vi "S4GUI_001.vi"() -> ()   [LabVIEW 2018] (continued)
            n3363 = call "Write target.vi"("error in (no error)"=w8575, "target"=0.0, "Optics in"=w8577) -> ("error out"=w8574:errorcluster, "Optics out"=w8578:refnum<class "Opt_Selector.lvclass">)  [unwired: 7 in]
            n3364 = call "Write target name.vi"("error in (no error)"=w8574, "target name"=w8568, "Optics in"=w8578) -> ("error out"=w8573:errorcluster, "Optics out"=w8579:refnum<class "Opt_Selector.lvclass">)  [unwired: 7 in]
            n3365 = call "Write CALW.vi"("error in (no error)"=w8573, "Opt_Selector.lvclass"=w8579, "Instrument in"=w8576) -> ("error out"=w8563:errorcluster, "Instrument out"=w8571:refnum<class "Instrument.lvclass">)  [unwired: 7 in]
            n3366 = property on="Calibrator Selector" class="Ring (strict)"(error in=w8563, "Value"=w8562, "DisabledEnum"=T7."Disabled and Grayed Out" ("Disabled")) -> (error out=w8565:errorcluster)  [unwired: 1 in, 1 out]
            n3367 = property on="Calibrator Selector" class="Ring (strict)"(error in=w8565, "RingText.Text"="OFF" ("Ring Text.Text")) -> (error out=w8564:errorcluster)  [unwired: 1 in, 1 out]
            n3368 = case shown="True" w8560 {
              tunnel: [u8 0 ("SHUTTER_MODE") w8582] -> w8561
              tunnel: w8559 -> [_ w8581]
              frame False {
                # "Fotom. & Async"
                # "Internal"
              }
              frame True {
                # "Ext. Start"
                # "Internal"
                # "Fotom. Sync. SEM exp mode"
                # "Fotom. Sync. COM exp mode"
                n3369 = Select(t=u8 0, s=w8581, f=u8 6 ("SHUTTER_MODE")) -> (s? t:f=w8582:u8)
              }
            }
          }
          frame Default {
            # "Polar. COM exp mode"
            # "Internal"
            # "Polar. SEM exp mode"
            # "Ext. Start"
            n3370 = Select(t=u8 0, s=w8588, f=u8 6 ("SHUTTER_MODE")) -> (s? t:f=w8585:u8)
          }
        }
        n3371 = call "Write Instrument.lvclass.vi"("error in (no error)"=w8236, "Instrument.lvclass"=w8319, "S4ACS_GUI in"=w8220) -> ("error out"=w8235:errorcluster, "S4ACS_GUI out"=w8224:refnum<class "S4GUI.lvclass">)  [unwired: 7 in]
        n3372 = call-dynamic "Read AcquisitionC.vi"("error in (no error)"=w8235, "S4ACS_GUI in"=w8224) -> ("error out"=w8246:errorcluster, "Acquisition.lvclass"=w8245:refnum<class "Acquisition.lvclass">)  [unwired: 7 in, 1 out]
        n3373 = call-dynamic "Read AcquisitionA.vi"("error in (no error)"=w8235, "S4ACS_GUI in"=w8224) -> ("error out"=w8249:errorcluster, "Acquisition.lvclass"=w8250:refnum<class "Acquisition.lvclass">)  [unwired: 7 in, 1 out]
        n3374 = call "Read AcquisitionB.vi"("error in (no error)"=w8235, "S4ACS_GUI in"=w8224) -> ("error out"=w8247:errorcluster, "Acquisition.lvclass"=w8248:refnum<class "Acquisition.lvclass">)  [unwired: 7 in, 1 out]
        n3375 = call-dynamic "Read AcquisitionD.vi"("error in (no error)"=w8235, "S4ACS_GUI in"=w8224) -> ("error out"=w8243:errorcluster, "Acquisition.lvclass"=w8244:refnum<class "Acquisition.lvclass">)  [unwired: 7 in, 1 out]
        n3376 = call "Read connection.vi"("error in (no error)"=w8246, "Server in"=w8245) -> ("error out"=w8252:errorcluster, "connection"=w8251:bool, "Server out"=w8253:refnum<class "Acquisition.lvclass">)  [unwired: 7 in]
        n3377 = call "Read connection.vi"("error in (no error)"=w8247, "Server in"=w8248) -> ("error out"=w8255:errorcluster, "connection"=w8254:bool, "Server out"=w8256:refnum<class "Acquisition.lvclass">)  [unwired: 7 in]
        n3378 = call "Read connection.vi"("error in (no error)"=w8243, "Server in"=w8244) -> ("error out"=w8232:errorcluster, "connection"=w8233:bool, "Server out"=w8234:refnum<class "Acquisition.lvclass">)  [unwired: 7 in]
        n3379 = call "Read connection.vi"("error in (no error)"=w8249, "Server in"=w8250) -> ("error out"=w8258:errorcluster, "connection"=w8257:bool, "Server out"=w8259:refnum<class "Acquisition.lvclass">)  [unwired: 7 in]
        n3380 = case shown="True" w8251 {
          tunnel: w8253 -> [w8426 w8431]
          tunnel: w8252 -> [w8425 w8430]
          tunnel: [w8426 w8429] -> w8238
          tunnel: [w8425 w8428] -> w8237
          tunnel: w8231 -> [_ w8427]
          frame False {
          }
          frame True {
            # "nome do arquivo .cfg"
            # "seção no arquivo .cfg"
            n3381 = call-dynamic "Read Channel.vi"("error in (no error)"=w8430, "Acquisition in"=w8431) -> ("error out"=w8435:errorcluster, "Channel.lvclass"=w8434:refnum<class "Channel.lvclass">, "Acquisition out"=w8433:refnum<class "Acquisition.lvclass">)  [unwired: 7 in]
            n3382 = call-dynamic "Read Interface.vi"("error in (no error)"=w8435, "Channel in"=w8434) -> ("error out"=w8442:errorcluster, "Interface.lvclass"=w8443:refnum<class "Interface.lvclass">, "Channel out"=w8432:refnum<class "Channel.lvclass">)  [unwired: 7 in]
            n3383 = call-dynamic "Get CCD_Config.vi"("error in (no error)"=w8442, "Interface in"=w8443) -> ("error out"=w8440:errorcluster, "output cluster"=w8439:T24, "Interface out"=w8444:refnum<class "Interface.lvclass">)  [unwired: 7 in]
            n3384 = Bundle By Name(cluster=w8439, "TRIGGER_MODE"=w8427) -> (w8441:T24)
            n3385 = call-dynamic "Set CCD_Config.vi"("error in (no error)"=w8440, "input cluster"=w8441, "Interface in"=w8444) -> ("error out"=w8438:errorcluster, "Interface out"=w8445:refnum<class "Interface.lvclass">)  [unwired: 7 in]
            n3386 = Flatten To String(anything=w8441, error in (no error)=w8438) -> (data string=w8436:string, error out=w8437:errorcluster)  [unwired: 2 in, 1 out]
            n3387 = call "Write flatted cluster.vi"("error in (no error)"=w8437, "flatted cluster"=w8436, "Interface in"=w8445) -> ("error out"=w8447:errorcluster, "Interface out"=w8446:refnum<class "Interface.lvclass">)  [unwired: 7 in]
            n3388 = call-dynamic "Write Interface.vi"("error in (no error)"=w8447, "Interface.lvclass"=w8446, "Channel in"=w8432) -> ("error out"=w8453:errorcluster, "Channel out"=w8454:refnum<class "Channel.lvclass">)  [unwired: 7 in]
            n3389 = call "Write section_name.vi"("error in (no error)"=w8453, "section_name"="CCD_ACS3", "Channel in"=w8454) -> ("error out"=w8451:errorcluster, "Channel out"=w8457:refnum<class "Channel.lvclass">)  [unwired: 7 in]
            n3390 = call-dynamic "save config.vi"("error in (no error)"=w8451, "file config"="lastsaved.cfg", "Channel in"=w8457) -> ("error out"=w8452:errorcluster, "Channel out"=w8458:refnum<class "Channel.lvclass">)  [unwired: 7 in]
            n3391 = call-dynamic "Read State Machine.vi"("error in (no error)"=w8452, "Device in"=w8458) -> ("error out"=w8448:errorcluster, "State Machine.lvclass"=w8460:refnum<class "State Machine.lvclass">, "Device out"=w8459:refnum<class "Channel.lvclass">)  [unwired: 7 in]
            n3392 = call-dynamic "Write State.vi"("error in (no error)"=w8448, "State"=60, "State Machine in"=w8460) -> ("error out"=w8449:errorcluster, "State Machine out"=w8461:refnum<class "State Machine.lvclass">)  [unwired: 7 in]
            n3393 = call-dynamic "Write State Machine.vi"("error in (no error)"=w8449, "State Machine.lvclass"=w8461, "Device in"=w8459) -> ("error out"=w8463:errorcluster, "Device out"=w8462:refnum<class "Channel.lvclass">)  [unwired: 7 in]
            n3394 = call-dynamic "Write Channel.vi"("error in (no error)"=w8463, "Channel.lvclass"=w8462, "Acquisition in"=w8433) -> ("error out"=w8428:errorcluster, "Acquisition out"=w8429:refnum<class "Acquisition.lvclass">)  [unwired: 7 in]
          }
        }
        n3395 = case shown="True" w8233 {
          tunnel: w8234 -> [w8387 w8392]
          tunnel: w8232 -> [w8386 w8391]
          tunnel: w8231 -> [_ w8390]
          tunnel: [w8387 w8389] -> w8230
          tunnel: [w8386 w8388] -> w8229
          frame False {
          }
          frame True {
            # "nome do arquivo .cfg"
            # "seção no arquivo .cfg"
            n3396 = call-dynamic "Read Channel.vi"("error in (no error)"=w8391, "Acquisition in"=w8392) -> ("error out"=w8421:errorcluster, "Channel.lvclass"=w8422:refnum<class "Channel.lvclass">, "Acquisition out"=w8423:refnum<class "Acquisition.lvclass">)  [unwired: 7 in]
            n3397 = call-dynamic "Read Interface.vi"("error in (no error)"=w8421, "Channel in"=w8422) -> ("error out"=w8414:errorcluster, "Interface.lvclass"=w8413:refnum<class "Interface.lvclass">, "Channel out"=w8424:refnum<class "Channel.lvclass">)  [unwired: 7 in]
            n3398 = call-dynamic "Get CCD_Config.vi"("error in (no error)"=w8414, "Interface in"=w8413) -> ("error out"=w8416:errorcluster, "output cluster"=w8417:T24, "Interface out"=w8412:refnum<class "Interface.lvclass">)  [unwired: 7 in]
            n3399 = Bundle By Name(cluster=w8417, "TRIGGER_MODE"=w8390) -> (w8415:T24)
            n3400 = call-dynamic "Set CCD_Config.vi"("error in (no error)"=w8416, "input cluster"=w8415, "Interface in"=w8412) -> ("error out"=w8418:errorcluster, "Interface out"=w8411:refnum<class "Interface.lvclass">)  [unwired: 7 in]
            n3401 = Flatten To String(anything=w8415, error in (no error)=w8418) -> (data string=w8420:string, error out=w8419:errorcluster)  [unwired: 2 in, 1 out]
            n3402 = call "Write flatted cluster.vi"("error in (no error)"=w8419, "flatted cluster"=w8420, "Interface in"=w8411) -> ("error out"=w8409:errorcluster, "Interface out"=w8410:refnum<class "Interface.lvclass">)  [unwired: 7 in]
            n3403 = call-dynamic "Write Interface.vi"("error in (no error)"=w8409, "Interface.lvclass"=w8410, "Channel in"=w8424) -> ("error out"=w8403:errorcluster, "Channel out"=w8402:refnum<class "Channel.lvclass">)  [unwired: 7 in]
            n3404 = call "Write section_name.vi"("error in (no error)"=w8403, "section_name"="CCD_ACS4", "Channel in"=w8402) -> ("error out"=w8405:errorcluster, "Channel out"=w8399:refnum<class "Channel.lvclass">)  [unwired: 7 in]
            n3405 = call-dynamic "save config.vi"("error in (no error)"=w8405, "file config"="lastsaved.cfg", "Channel in"=w8399) -> ("error out"=w8404:errorcluster, "Channel out"=w8398:refnum<class "Channel.lvclass">)  [unwired: 7 in]
            n3406 = call-dynamic "Read State Machine.vi"("error in (no error)"=w8404, "Device in"=w8398) -> ("error out"=w8408:errorcluster, "State Machine.lvclass"=w8396:refnum<class "State Machine.lvclass">, "Device out"=w8397:refnum<class "Channel.lvclass">)  [unwired: 7 in]
            n3407 = call-dynamic "Write State.vi"("error in (no error)"=w8408, "State"=60, "State Machine in"=w8396) -> ("error out"=w8407:errorcluster, "State Machine out"=w8395:refnum<class "State Machine.lvclass">)  [unwired: 7 in]
            n3408 = call-dynamic "Write State Machine.vi"("error in (no error)"=w8407, "State Machine.lvclass"=w8395, "Device in"=w8397) -> ("error out"=w8393:errorcluster, "Device out"=w8394:refnum<class "Channel.lvclass">)  [unwired: 7 in]
            n3409 = call-dynamic "Write Channel.vi"("error in (no error)"=w8393, "Channel.lvclass"=w8394, "Acquisition in"=w8423) -> ("error out"=w8388:errorcluster, "Acquisition out"=w8389:refnum<class "Acquisition.lvclass">)  [unwired: 7 in]
          }
        }
        n3410 = case shown="True" w8254 {
          tunnel: w8256 -> [w8465 w8470]
          tunnel: w8255 -> [w8464 w8469]
          tunnel: [w8465 w8468] -> w8240
          tunnel: [w8464 w8467] -> w8239
          tunnel: w8231 -> [_ w8466]
          frame False {
          }
          frame True {
            # "nome do arquivo .cfg"
            # "seção no arquivo .cfg"
            n3411 = call-dynamic "Read Channel.vi"("error in (no error)"=w8469, "Acquisition in"=w8470) -> ("error out"=w8474:errorcluster, "Channel.lvclass"=w8473:refnum<class "Channel.lvclass">, "Acquisition out"=w8472:refnum<class "Acquisition.lvclass">)  [unwired: 7 in]
            n3412 = call-dynamic "Read Interface.vi"("error in (no error)"=w8474, "Channel in"=w8473) -> ("error out"=w8481:errorcluster, "Interface.lvclass"=w8482:refnum<class "Interface.lvclass">, "Channel out"=w8471:refnum<class "Channel.lvclass">)  [unwired: 7 in]
            n3413 = call-dynamic "Get CCD_Config.vi"("error in (no error)"=w8481, "Interface in"=w8482) -> ("error out"=w8479:errorcluster, "output cluster"=w8478:T24, "Interface out"=w8483:refnum<class "Interface.lvclass">)  [unwired: 7 in]
            n3414 = Bundle By Name(cluster=w8478, "TRIGGER_MODE"=w8466) -> (w8480:T24)
            n3415 = call-dynamic "Set CCD_Config.vi"("error in (no error)"=w8479, "input cluster"=w8480, "Interface in"=w8483) -> ("error out"=w8477:errorcluster, "Interface out"=w8484:refnum<class "Interface.lvclass">)  [unwired: 7 in]
            n3416 = Flatten To String(anything=w8480, error in (no error)=w8477) -> (data string=w8475:string, error out=w8476:errorcluster)  [unwired: 2 in, 1 out]
            n3417 = call "Write flatted cluster.vi"("error in (no error)"=w8476, "flatted cluster"=w8475, "Interface in"=w8484) -> ("error out"=w8486:errorcluster, "Interface out"=w8485:refnum<class "Interface.lvclass">)  [unwired: 7 in]
            n3418 = call-dynamic "Write Interface.vi"("error in (no error)"=w8486, "Interface.lvclass"=w8485, "Channel in"=w8471) -> ("error out"=w8492:errorcluster, "Channel out"=w8493:refnum<class "Channel.lvclass">)  [unwired: 7 in]
            n3419 = call "Write section_name.vi"("error in (no error)"=w8492, "section_name"="CCD_ACS2", "Channel in"=w8493) -> ("error out"=w8490:errorcluster, "Channel out"=w8496:refnum<class "Channel.lvclass">)  [unwired: 7 in]
            n3420 = call-dynamic "save config.vi"("error in (no error)"=w8490, "file config"="lastsaved.cfg", "Channel in"=w8496) -> ("error out"=w8491:errorcluster, "Channel out"=w8497:refnum<class "Channel.lvclass">)  [unwired: 7 in]
            n3421 = call-dynamic "Read State Machine.vi"("error in (no error)"=w8491, "Device in"=w8497) -> ("error out"=w8487:errorcluster, "State Machine.lvclass"=w8499:refnum<class "State Machine.lvclass">, "Device out"=w8498:refnum<class "Channel.lvclass">)  [unwired: 7 in]
            n3422 = call-dynamic "Write State.vi"("error in (no error)"=w8487, "State"=60, "State Machine in"=w8499) -> ("error out"=w8488:errorcluster, "State Machine out"=w8500:refnum<class "State Machine.lvclass">)  [unwired: 7 in]
            n3423 = call-dynamic "Write State Machine.vi"("error in (no error)"=w8488, "State Machine.lvclass"=w8500, "Device in"=w8498) -> ("error out"=w8502:errorcluster, "Device out"=w8501:refnum<class "Channel.lvclass">)  [unwired: 7 in]
            n3424 = call-dynamic "Write Channel.vi"("error in (no error)"=w8502, "Channel.lvclass"=w8501, "Acquisition in"=w8472) -> ("error out"=w8467:errorcluster, "Acquisition out"=w8468:refnum<class "Acquisition.lvclass">)  [unwired: 7 in]
          }
        }
        n3425 = case shown="True" w8257 {
          tunnel: [w8503 w8537] -> w8241
          tunnel: [w8504 w8536] -> w8242
          tunnel: w8259 -> [w8504 w8507]
          tunnel: w8258 -> [w8503 w8506]
          tunnel: w8231 -> [_ w8505]
          frame False {
          }
          frame True {
            # "nome do arquivo .cfg"
            # "seção no arquivo .cfg"
            n3426 = call-dynamic "Read Channel.vi"("error in (no error)"=w8506, "Acquisition in"=w8507) -> ("error out"=w8538:errorcluster, "Channel.lvclass"=w8539:refnum<class "Channel.lvclass">, "Acquisition out"=w8540:refnum<class "Acquisition.lvclass">)  [unwired: 7 in]
            n3427 = call-dynamic "Read Interface.vi"("error in (no error)"=w8538, "Channel in"=w8539) -> ("error out"=w8529:errorcluster, "Interface.lvclass"=w8528:refnum<class "Interface.lvclass">, "Channel out"=w8541:refnum<class "Channel.lvclass">)  [unwired: 7 in]
            n3428 = call-dynamic "Get CCD_Config.vi"("error in (no error)"=w8529, "Interface in"=w8528) -> ("error out"=w8531:errorcluster, "output cluster"=w8532:T24, "Interface out"=w8527:refnum<class "Interface.lvclass">)  [unwired: 7 in]
            n3429 = Bundle By Name(cluster=w8532, "TRIGGER_MODE"=w8505) -> (w8530:T24)
            n3430 = call-dynamic "Set CCD_Config.vi"("error in (no error)"=w8531, "input cluster"=w8530, "Interface in"=w8527) -> ("error out"=w8533:errorcluster, "Interface out"=w8526:refnum<class "Interface.lvclass">)  [unwired: 7 in]
            n3431 = Flatten To String(anything=w8530, error in (no error)=w8533) -> (data string=w8535:string, error out=w8534:errorcluster)  [unwired: 2 in, 1 out]
            n3432 = call "Write flatted cluster.vi"("error in (no error)"=w8534, "flatted cluster"=w8535, "Interface in"=w8526) -> ("error out"=w8524:errorcluster, "Interface out"=w8525:refnum<class "Interface.lvclass">)  [unwired: 7 in]
            n3433 = call-dynamic "Write Interface.vi"("error in (no error)"=w8524, "Interface.lvclass"=w8525, "Channel in"=w8541) -> ("error out"=w8519:errorcluster, "Channel out"=w8518:refnum<class "Channel.lvclass">)  [unwired: 7 in]
            n3434 = call "Write section_name.vi"("error in (no error)"=w8519, "section_name"="CCD_ACS1", "Channel in"=w8518) -> ("error out"=w8520:errorcluster, "Channel out"=w8515:refnum<class "Channel.lvclass">)  [unwired: 7 in]
            n3435 = call-dynamic "save config.vi"("error in (no error)"=w8520, "file config"="lastsaved.cfg", "Channel in"=w8515) -> ("error out"=w8508:errorcluster, "Channel out"=w8509:refnum<class "Channel.lvclass">)  [unwired: 7 in]
            n3436 = call-dynamic "Read State Machine.vi"("error in (no error)"=w8508, "Device in"=w8509) -> ("error out"=w8523:errorcluster, "State Machine.lvclass"=w8513:refnum<class "State Machine.lvclass">, "Device out"=w8514:refnum<class "Channel.lvclass">)  [unwired: 7 in]
            n3437 = call-dynamic "Write State.vi"("error in (no error)"=w8523, "State"=60, "State Machine in"=w8513) -> ("error out"=w8522:errorcluster, "State Machine out"=w8512:refnum<class "State Machine.lvclass">)  [unwired: 7 in]
            n3438 = call-dynamic "Write State Machine.vi"("error in (no error)"=w8522, "State Machine.lvclass"=w8512, "Device in"=w8514) -> ("error out"=w8510:errorcluster, "Device out"=w8511:refnum<class "Channel.lvclass">)  [unwired: 7 in]
            n3439 = call-dynamic "Write Channel.vi"("error in (no error)"=w8510, "Channel.lvclass"=w8511, "Acquisition in"=w8540) -> ("error out"=w8537:errorcluster, "Acquisition out"=w8536:refnum<class "Acquisition.lvclass">)  [unwired: 7 in]
          }
        }
        n3440 = call-dynamic "Write AcquisitionA.vi"("error in (no error)"=w8241, "Acquisition.lvclass"=w8242, "S4ACS_GUI in"=w8224) -> ("error out"=w8228:errorcluster, "S4ACS_GUI out"=w8223:refnum<class "S4GUI.lvclass">)  [unwired: 7 in]
        n3441 = call "Write AcquisitionB.vi"("error in (no error)"=w8239, "Acquisition.lvclass"=w8240, "S4ACS_GUI in"=w8223) -> ("error out"=w8227:errorcluster, "S4ACS_GUI out"=w8222:refnum<class "S4GUI.lvclass">)  [unwired: 7 in]
        n3442 = call-dynamic "Write AcquisitionC.vi"("error in (no error)"=w8237, "Acquisition.lvclass"=w8238, "S4ACS_GUI in"=w8222) -> ("error out"=w8226:errorcluster, "S4ACS_GUI out"=w8221:refnum<class "S4GUI.lvclass">)  [unwired: 7 in]
        n3443 = call-dynamic "Write AcquisitionD.vi"("error in (no error)"=w8229, "Acquisition.lvclass"=w8230, "S4ACS_GUI in"=w8221) -> ("error out"=w8225:errorcluster, "S4ACS_GUI out"=w8204:refnum<class "S4GUI.lvclass">)  [unwired: 7 in]
        n3444 = Merge Errors(w8228, w8227, w8226, w8225) -> (w8201:errorcluster)
        n3445 = call "Read Instrument.lvclass.vi"("error in (no error)"=w8201, "S4ACS_GUI in"=w8204) -> ("error out"=w8209:errorcluster, "Instrument.lvclass"=w8208:refnum<class "Instrument.lvclass">, "S4ACS_GUI out"=w8205:refnum<class "S4GUI.lvclass">)  [unwired: 7 in]
        n3446 = call "Read ASEL.vi"("error in (no error)"=w8209, "Instrument in"=w8208) -> ("error out"=w8217:errorcluster, "Opt_Selector.lvclass"=w8216:refnum<class "Opt_Selector.lvclass">, "Instrument out"=w8215:refnum<class "Instrument.lvclass">)  [unwired: 7 in]
        n3447 = call "Read target name.vi"("error in (no error)"=w8217, "Optics in"=w8216) -> ("error out"=w8213:errorcluster, "target name"=w8212:string, "Optics out"=w8214:refnum<class "Opt_Selector.lvclass">)  [unwired: 7 in]
        n3448 = call "Write ASEL.vi"("error in (no error)"=w8213, "Opt_Selector.lvclass"=w8214, "Instrument in"=w8215) -> ("error out"=w8211:errorcluster, "Instrument out"=w8207:refnum<class "Instrument.lvclass">)  [unwired: 7 in]
        n3449 = case shown="\"ON\"" w8212 {
          tunnel: w8211 -> [w8362 w8373]
          tunnel: [w8362 w8369] -> w8210
          tunnel: w8207 -> [w8361 w8374]
          tunnel: [w8361 w8370] -> w8206
          frame Default {
          }
          frame "ON" {
            n3450 = call "Read WPROT.vi"("error in (no error)"=w8373, "Instrument in"=w8374) -> ("error out"=w8365:errorcluster, "Opt_Selector.lvclass"=w8372:refnum<class "Opt_Selector.lvclass">, "Instrument out"=w8371:refnum<class "Instrument.lvclass">)  [unwired: 7 in]
            n3451 = call-dynamic "Read sequencia.vi"("error in (no error)"=w8365, "Opt_Selector in"=w8372) -> ("error out"=w8364:errorcluster, "sequencia"=w8368:u16, "Opt_Selector out"=w8367:refnum<class "Opt_Selector.lvclass">)  [unwired: 7 in]
            n3452 = case shown="0" w8368 {
              tunnel: w8367 -> [w8376 w8385]
              tunnel: [w8376 w8381] -> w8366
              tunnel: w8364 -> [w8375 w8384]
              tunnel: [w8375 w8379] -> w8363
              frame Default {
              }
              frame 0 {
                n3453 = call-dynamic "Write sequencia.vi"("error in (no error)"=w8384, "sequencia"=u16 1, "Opt_Selector in"=w8385) -> ("error out"=w8380:errorcluster, "Opt_Selector out"=w8382:refnum<class "Opt_Selector.lvclass">)  [unwired: 7 in]
                n3454 = local write "P0"(TRUE ("P0")) -> ()
                n3455 = call-dynamic "Write sequencia_ant.vi"("error in (no error)"=w8380, "sequencia_ant"=u16 1, "Opt_Selector in"=w8382) -> ("error out"=w8379:errorcluster, "Opt_Selector out"=w8381:refnum<class "Opt_Selector.lvclass">)  [unwired: 7 in]
              }
            }
            n3456 = call "Write WPROT.vi"("error in (no error)"=w8363, "Opt_Selector.lvclass"=w8366, "Instrument in"=w8371) -> ("error out"=w8369:errorcluster, "Instrument out"=w8370:refnum<class "Instrument.lvclass">)  [unwired: 7 in]
          }
        }
        n3457 = call "Write Instrument.lvclass.vi"("error in (no error)"=w8210, "Instrument.lvclass"=w8206, "S4ACS_GUI in"=w8205) -> ("error out"=w8202:errorcluster, "S4ACS_GUI out"=w8203:refnum<class "S4GUI.lvclass">)  [unwired: 7 in]
      }
      event "Init mode": Value Change {
        n3458 = event-data() -> ()  [unwired: 1 in, 4 out]
        n3459 = call-dynamic "Read Obs_state.vi"("error in (no error)"=w8597, "S4ACS_GUI in"=w8598) -> ("error out"=w8591:errorcluster, "Obs_state"=w8593:u32, "S4ACS_GUI out"=w8594:refnum<class "S4GUI.lvclass">)  [unwired: 7 in]
        n3460 = In Range and Coerce(upper limit=u32 226, x=w8593, lower limit=u32 220 ("upper limit")) -> (In Range?=w8592:bool)  [unwired: 1 out]
        n3461 = case shown="False" w8592 {
          tunnel: [w8604 w8612] -> w8600
          tunnel: [w8603 w8610] -> w8599
          tunnel: w8591 -> [w8602 w8611]
          tunnel: w8594 -> [w8601 w8613]
          frame False {
            n3462 = call-dynamic "Write sync.vi"("error in (no error)"=w8602, "sync"=TRUE, "S4ACS_GUI in"=w8601) -> ("error out"=w8606:errorcluster, "S4ACS_GUI out"=w8605:refnum<class "S4GUI.lvclass">)  [unwired: 7 in]
            n3463 = call-dynamic "Write Obs_state.vi"("error in (no error)"=w8606, "Obs_state"=u32 220, "S4ACS_GUI in"=w8605) -> ("error out"=w8603:errorcluster, "S4ACS_GUI out"=w8604:refnum<class "S4GUI.lvclass">)  [unwired: 7 in]
          }
          frame True {
            n3464 = call-dynamic "Write Obs_state.vi"("error in (no error)"=w8611, "Obs_state"=u32 0, "S4ACS_GUI in"=w8613) -> ("error out"=w8610:errorcluster, "S4ACS_GUI out"=w8612:refnum<class "S4GUI.lvclass">)  [unwired: 7 in]
          }
        }
      }
      event "Set PCS": Value Change {
        n3465 = event-data() -> ()  [unwired: 1 in, 4 out]
        n3466 = call "Read Instrument.lvclass.vi"("error in (no error)"=w8632, "S4ACS_GUI in"=w8633) -> ("error out"=w8630:errorcluster, "Instrument.lvclass"=w8631:refnum<class "Instrument.lvclass">, "S4ACS_GUI out"=w8619:refnum<class "S4GUI.lvclass">)  [unwired: 7 in]
        n3467 = call "Read CALW.vi"("error in (no error)"=w8630, "Instrument in"=w8631) -> ("error out"=w8627:errorcluster, "Opt_Selector.lvclass"=w8629:refnum<class "Opt_Selector.lvclass">, "Instrument out"=w8621:refnum<class "Instrument.lvclass">)  [unwired: 7 in]
        n3468 = call-dynamic "Read State Machine.vi"("error in (no error)"=w8627, "Device in"=w8629) -> ("error out"=w8626:errorcluster, "State Machine.lvclass"=w8617:refnum<class "State Machine.lvclass">, "Device out"=w8623:refnum<class "Opt_Selector.lvclass">)  [unwired: 7 in]
        n3469 = call "Next State.vi"("error in (no error)"=w8626, "New_State"=1, "State Machine in"=w8617) -> ("error out"=w8625:errorcluster, "State Machine out"=w8624:refnum<class "State Machine.lvclass">)  [unwired: 7 in]
        n3470 = call-dynamic "Write State Machine.vi"("error in (no error)"=w8625, "State Machine.lvclass"=w8624, "Device in"=w8623) -> ("error out"=w8620:errorcluster, "Device out"=w8622:refnum<class "Opt_Selector.lvclass">)  [unwired: 7 in]
        n3471 = call "Write CALW.vi"("error in (no error)"=w8620, "Opt_Selector.lvclass"=w8622, "Instrument in"=w8621) -> ("error out"=w8615:errorcluster, "Instrument out"=w8616:refnum<class "Instrument.lvclass">)  [unwired: 7 in]
        n3472 = call "Write Instrument.lvclass.vi"("error in (no error)"=w8615, "Instrument.lvclass"=w8616, "S4ACS_GUI in"=w8619) -> ("error out"=w8618:errorcluster, "S4ACS_GUI out"=w8614:refnum<class "S4GUI.lvclass">)  [unwired: 7 in]
      }
      event "WPSEL_stop": Value Change {
        n3473 = event-data() -> ()  [unwired: 1 in, 4 out]
        n3474 = call "Read Instrument.lvclass.vi"("error in (no error)"=w8652, "S4ACS_GUI in"=w8653) -> ("error out"=w8650:errorcluster, "Instrument.lvclass"=w8651:refnum<class "Instrument.lvclass">, "S4ACS_GUI out"=w8637:refnum<class "S4GUI.lvclass">)  [unwired: 7 in]
        n3475 = call "Read WPSEL.vi"("error in (no error)"=w8650, "Instrument in"=w8651) -> ("error out"=w8646:errorcluster, "Opt_Selector.lvclass"=w8649:refnum<class "Opt_Selector.lvclass">, "Instrument out"=w8640:refnum<class "Instrument.lvclass">)  [unwired: 7 in]
        n3476 = call-dynamic "Read State Machine.vi"("error in (no error)"=w8646, "Device in"=w8649) -> ("error out"=w8645:errorcluster, "State Machine.lvclass"=w8648:refnum<class "State Machine.lvclass">, "Device out"=w8642:refnum<class "Opt_Selector.lvclass">)  [unwired: 7 in]
        n3477 = call "Next State.vi"("error in (no error)"=w8645, "New_State"=10, "State Machine in"=w8648) -> ("error out"=w8644:errorcluster, "State Machine out"=w8643:refnum<class "State Machine.lvclass">)  [unwired: 7 in]
        n3478 = call-dynamic "Write State Machine.vi"("error in (no error)"=w8644, "State Machine.lvclass"=w8643, "Device in"=w8642) -> ("error out"=w8639:errorcluster, "Device out"=w8641:refnum<class "Opt_Selector.lvclass">)  [unwired: 7 in]
        n3479 = call "Write WPSEL.vi"("error in (no error)"=w8639, "Opt_Selector.lvclass"=w8641, "Instrument in"=w8640) -> ("error out"=w8636:errorcluster, "Instrument out"=w8638:refnum<class "Instrument.lvclass">)  [unwired: 7 in]
        n3480 = call "Write Instrument.lvclass.vi"("error in (no error)"=w8636, "Instrument.lvclass"=w8638, "S4ACS_GUI in"=w8637) -> ("error out"=w8635:errorcluster, "S4ACS_GUI out"=w8634:refnum<class "S4GUI.lvclass">)  [unwired: 7 in]
      }
      event "WPSEL_init": Value Change {
        n3481 = event-data() -> ()  [unwired: 1 in, 4 out]
        n3482 = call "Read Instrument.lvclass.vi"("error in (no error)"=w8672, "S4ACS_GUI in"=w8673) -> ("error out"=w8670:errorcluster, "Instrument.lvclass"=w8671:refnum<class "Instrument.lvclass">, "S4ACS_GUI out"=w8657:refnum<class "S4GUI.lvclass">)  [unwired: 7 in]
        n3483 = call "Read WPSEL.vi"("error in (no error)"=w8670, "Instrument in"=w8671) -> ("error out"=w8666:errorcluster, "Opt_Selector.lvclass"=w8669:refnum<class "Opt_Selector.lvclass">, "Instrument out"=w8660:refnum<class "Instrument.lvclass">)  [unwired: 7 in]
        n3484 = call-dynamic "Read State Machine.vi"("error in (no error)"=w8666, "Device in"=w8669) -> ("error out"=w8665:errorcluster, "State Machine.lvclass"=w8668:refnum<class "State Machine.lvclass">, "Device out"=w8662:refnum<class "Opt_Selector.lvclass">)  [unwired: 7 in]
        n3485 = call "Next State.vi"("error in (no error)"=w8665, "New_State"=30, "State Machine in"=w8668) -> ("error out"=w8664:errorcluster, "State Machine out"=w8663:refnum<class "State Machine.lvclass">)  [unwired: 7 in]
        n3486 = call-dynamic "Write State Machine.vi"("error in (no error)"=w8664, "State Machine.lvclass"=w8663, "Device in"=w8662) -> ("error out"=w8659:errorcluster, "Device out"=w8661:refnum<class "Opt_Selector.lvclass">)  [unwired: 7 in]
        n3487 = call "Write WPSEL.vi"("error in (no error)"=w8659, "Opt_Selector.lvclass"=w8661, "Instrument in"=w8660) -> ("error out"=w8656:errorcluster, "Instrument out"=w8658:refnum<class "Instrument.lvclass">)  [unwired: 7 in]
        n3488 = call "Write Instrument.lvclass.vi"("error in (no error)"=w8656, "Instrument.lvclass"=w8658, "S4ACS_GUI in"=w8657) -> ("error out"=w8655:errorcluster, "S4ACS_GUI out"=w8654:refnum<class "S4GUI.lvclass">)  [unwired: 7 in]
      }
      event "GMIR_target": Value Change {
        n3489 = event-data() -> ("NewVal"=w8683:dbl)  [unwired: 1 in, 3 out]
        n3490 = call "Read Instrument.lvclass.vi"("error in (no error)"=w8687, "S4ACS_GUI in"=w8688) -> ("error out"=w8685:errorcluster, "Instrument.lvclass"=w8686:refnum<class "Instrument.lvclass">, "S4ACS_GUI out"=w8677:refnum<class "S4GUI.lvclass">)  [unwired: 7 in]
        n3491 = call "Read GMIR.vi"("error in (no error)"=w8685, "Instrument in"=w8686) -> ("error out"=w8682:errorcluster, "Opt_Continuous.lvclass"=w8684:refnum<class "Opt_Continuous.lvclass">, "Instrument out"=w8680:refnum<class "Instrument.lvclass">)  [unwired: 7 in]
        n3492 = call "Write target.vi"("error in (no error)"=w8682, "target"=w8683, "Optics in"=w8684) -> ("error out"=w8679:errorcluster, "Optics out"=w8681:refnum<class "Opt_Continuous.lvclass">)  [unwired: 7 in]
        n3493 = call "Write GMIR.vi"("error in (no error)"=w8679, "Opt_Continuous.lvclass"=w8681, "Instrument in"=w8680) -> ("error out"=w8676:errorcluster, "Instrument out"=w8678:refnum<class "Instrument.lvclass">)  [unwired: 7 in]
        n3494 = call "Write Instrument.lvclass.vi"("error in (no error)"=w8676, "Instrument.lvclass"=w8678, "S4ACS_GUI in"=w8677) -> ("error out"=w8675:errorcluster, "S4ACS_GUI out"=w8674:refnum<class "S4GUI.lvclass">)  [unwired: 7 in]
      }
      event "GMIR_set": Value Change {
        n3495 = event-data() -> ()  [unwired: 1 in, 4 out]
        n3496 = call "Read Instrument.lvclass.vi"("error in (no error)"=w8707, "S4ACS_GUI in"=w8708) -> ("error out"=w8705:errorcluster, "Instrument.lvclass"=w8706:refnum<class "Instrument.lvclass">, "S4ACS_GUI out"=w8694:refnum<class "S4GUI.lvclass">)  [unwired: 7 in]
        n3497 = call "Read GMIR.vi"("error in (no error)"=w8705, "Instrument in"=w8706) -> ("error out"=w8702:errorcluster, "Opt_Continuous.lvclass"=w8704:refnum<class "Opt_Continuous.lvclass">, "Instrument out"=w8696:refnum<class "Instrument.lvclass">)  [unwired: 7 in]
        n3498 = call-dynamic "Read State Machine.vi"("error in (no error)"=w8702, "Device in"=w8704) -> ("error out"=w8701:errorcluster, "State Machine.lvclass"=w8692:refnum<class "State Machine.lvclass">, "Device out"=w8698:refnum<class "Opt_Continuous.lvclass">)  [unwired: 7 in]
        n3499 = call "Next State.vi"("error in (no error)"=w8701, "New_State"=1, "State Machine in"=w8692) -> ("error out"=w8700:errorcluster, "State Machine out"=w8699:refnum<class "State Machine.lvclass">)  [unwired: 7 in]
        n3500 = call-dynamic "Write State Machine.vi"("error in (no error)"=w8700, "State Machine.lvclass"=w8699, "Device in"=w8698) -> ("error out"=w8695:errorcluster, "Device out"=w8697:refnum<class "Opt_Continuous.lvclass">)  [unwired: 7 in]
        n3501 = call "Write GMIR.vi"("error in (no error)"=w8695, "Opt_Continuous.lvclass"=w8697, "Instrument in"=w8696) -> ("error out"=w8689:errorcluster, "Instrument out"=w8690:refnum<class "Instrument.lvclass">)  [unwired: 7 in]
        n3502 = call "Write Instrument.lvclass.vi"("error in (no error)"=w8689, "Instrument.lvclass"=w8690, "S4ACS_GUI in"=w8694) -> ("error out"=w8693:errorcluster, "S4ACS_GUI out"=w8691:refnum<class "S4GUI.lvclass">)  [unwired: 7 in]
      }
      event "GMIR_stop": Value Change {
        n3503 = event-data() -> ()  [unwired: 1 in, 4 out]
        n3504 = call "Read Instrument.lvclass.vi"("error in (no error)"=w8727, "S4ACS_GUI in"=w8728) -> ("error out"=w8725:errorcluster, "Instrument.lvclass"=w8726:refnum<class "Instrument.lvclass">, "S4ACS_GUI out"=w8712:refnum<class "S4GUI.lvclass">)  [unwired: 7 in]
        n3505 = call "Read GMIR.vi"("error in (no error)"=w8725, "Instrument in"=w8726) -> ("error out"=w8721:errorcluster, "Opt_Continuous.lvclass"=w8724:refnum<class "Opt_Continuous.lvclass">, "Instrument out"=w8715:refnum<class "Instrument.lvclass">)  [unwired: 7 in]
        n3506 = call-dynamic "Read State Machine.vi"("error in (no error)"=w8721, "Device in"=w8724) -> ("error out"=w8720:errorcluster, "State Machine.lvclass"=w8723:refnum<class "State Machine.lvclass">, "Device out"=w8717:refnum<class "Opt_Continuous.lvclass">)  [unwired: 7 in]
        n3507 = call "Next State.vi"("error in (no error)"=w8720, "New_State"=10, "State Machine in"=w8723) -> ("error out"=w8719:errorcluster, "State Machine out"=w8718:refnum<class "State Machine.lvclass">)  [unwired: 7 in]
        n3508 = call-dynamic "Write State Machine.vi"("error in (no error)"=w8719, "State Machine.lvclass"=w8718, "Device in"=w8717) -> ("error out"=w8714:errorcluster, "Device out"=w8716:refnum<class "Opt_Continuous.lvclass">)  [unwired: 7 in]
        n3509 = call "Write GMIR.vi"("error in (no error)"=w8714, "Opt_Continuous.lvclass"=w8716, "Instrument in"=w8715) -> ("error out"=w8711:errorcluster, "Instrument out"=w8713:refnum<class "Instrument.lvclass">)  [unwired: 7 in]
        n3510 = call "Write Instrument.lvclass.vi"("error in (no error)"=w8711, "Instrument.lvclass"=w8713, "S4ACS_GUI in"=w8712) -> ("error out"=w8710:errorcluster, "S4ACS_GUI out"=w8709:refnum<class "S4GUI.lvclass">)  [unwired: 7 in]
      }
      event "GMIR_init": Value Change {
        n3511 = event-data() -> ()  [unwired: 1 in, 4 out]
        n3512 = call "Read Instrument.lvclass.vi"("error in (no error)"=w8747, "S4ACS_GUI in"=w8748) -> ("error out"=w8745:errorcluster, "Instrument.lvclass"=w8746:refnum<class "Instrument.lvclass">, "S4ACS_GUI out"=w8732:refnum<class "S4GUI.lvclass">)  [unwired: 7 in]
        n3513 = call "Read GMIR.vi"("error in (no error)"=w8745, "Instrument in"=w8746) -> ("error out"=w8741:errorcluster, "Opt_Continuous.lvclass"=w8744:refnum<class "Opt_Continuous.lvclass">, "Instrument out"=w8735:refnum<class "Instrument.lvclass">)  [unwired: 7 in]
        n3514 = call-dynamic "Read State Machine.vi"("error in (no error)"=w8741, "Device in"=w8744) -> ("error out"=w8740:errorcluster, "State Machine.lvclass"=w8743:refnum<class "State Machine.lvclass">, "Device out"=w8737:refnum<class "Opt_Continuous.lvclass">)  [unwired: 7 in]
        n3515 = call "Next State.vi"("error in (no error)"=w8740, "New_State"=30, "State Machine in"=w8743) -> ("error out"=w8739:errorcluster, "State Machine out"=w8738:refnum<class "State Machine.lvclass">)  [unwired: 7 in]
        n3516 = call-dynamic "Write State Machine.vi"("error in (no error)"=w8739, "State Machine.lvclass"=w8738, "Device in"=w8737) -> ("error out"=w8734:errorcluster, "Device out"=w8736:refnum<class "Opt_Continuous.lvclass">)  [unwired: 7 in]
        n3517 = call "Write GMIR.vi"("error in (no error)"=w8734, "Opt_Continuous.lvclass"=w8736, "Instrument in"=w8735) -> ("error out"=w8731:errorcluster, "Instrument out"=w8733:refnum<class "Instrument.lvclass">)  [unwired: 7 in]
        n3518 = call "Write Instrument.lvclass.vi"("error in (no error)"=w8731, "Instrument.lvclass"=w8733, "S4ACS_GUI in"=w8732) -> ("error out"=w8730:errorcluster, "S4ACS_GUI out"=w8729:refnum<class "S4GUI.lvclass">)  [unwired: 7 in]
      }
      event "GFOC_target": Value Change {
        n3519 = event-data() -> ("NewVal"=w8758:dbl)  [unwired: 1 in, 3 out]
        n3520 = call "Read Instrument.lvclass.vi"("error in (no error)"=w8762, "S4ACS_GUI in"=w8763) -> ("error out"=w8760:errorcluster, "Instrument.lvclass"=w8761:refnum<class "Instrument.lvclass">, "S4ACS_GUI out"=w8752:refnum<class "S4GUI.lvclass">)  [unwired: 7 in]
        n3521 = call "Read GFOC.vi"("error in (no error)"=w8760, "Instrument in"=w8761) -> ("error out"=w8757:errorcluster, "Opt_Continuous.lvclass"=w8759:refnum<class "Opt_Continuous.lvclass">, "Instrument out"=w8755:refnum<class "Instrument.lvclass">)  [unwired: 7 in]
        n3522 = call "Write target.vi"("error in (no error)"=w8757, "target"=w8758, "Optics in"=w8759) -> ("error out"=w8754:errorcluster, "Optics out"=w8756:refnum<class "Opt_Continuous.lvclass">)  [unwired: 7 in]
        n3523 = call "Write GFOC.vi"("error in (no error)"=w8754, "Opt_Continuous.lvclass"=w8756, "Instrument in"=w8755) -> ("error out"=w8751:errorcluster, "Instrument out"=w8753:refnum<class "Instrument.lvclass">)  [unwired: 7 in]
        n3524 = call "Write Instrument.lvclass.vi"("error in (no error)"=w8751, "Instrument.lvclass"=w8753, "S4ACS_GUI in"=w8752) -> ("error out"=w8750:errorcluster, "S4ACS_GUI out"=w8749:refnum<class "S4GUI.lvclass">)  [unwired: 7 in]
      }
      event "GFOC_set": Value Change {
        n3525 = event-data() -> ()  [unwired: 1 in, 4 out]
        n3526 = call "Read Instrument.lvclass.vi"("error in (no error)"=w8782, "S4ACS_GUI in"=w8783) -> ("error out"=w8780:errorcluster, "Instrument.lvclass"=w8781:refnum<class "Instrument.lvclass">, "S4ACS_GUI out"=w8768:refnum<class "S4GUI.lvclass">)  [unwired: 7 in]
        n3527 = call "Read GFOC.vi"("error in (no error)"=w8780, "Instrument in"=w8781) -> ("error out"=w8777:errorcluster, "Opt_Continuous.lvclass"=w8779:refnum<class "Opt_Continuous.lvclass">, "Instrument out"=w8771:refnum<class "Instrument.lvclass">)  [unwired: 7 in]
        n3528 = call-dynamic "Read State Machine.vi"("error in (no error)"=w8777, "Device in"=w8779) -> ("error out"=w8776:errorcluster, "State Machine.lvclass"=w8765:refnum<class "State Machine.lvclass">, "Device out"=w8773:refnum<class "Opt_Continuous.lvclass">)  [unwired: 7 in]
        n3529 = call "Next State.vi"("error in (no error)"=w8776, "New_State"=1, "State Machine in"=w8765) -> ("error out"=w8775:errorcluster, "State Machine out"=w8774:refnum<class "State Machine.lvclass">)  [unwired: 7 in]
        n3530 = call-dynamic "Write State Machine.vi"("error in (no error)"=w8775, "State Machine.lvclass"=w8774, "Device in"=w8773) -> ("error out"=w8770:errorcluster, "Device out"=w8772:refnum<class "Opt_Continuous.lvclass">)  [unwired: 7 in]
        n3531 = call "Write GFOC.vi"("error in (no error)"=w8770, "Opt_Continuous.lvclass"=w8772, "Instrument in"=w8771) -> ("error out"=w8767:errorcluster, "Instrument out"=w8769:refnum<class "Instrument.lvclass">)  [unwired: 7 in]
        n3532 = call "Write Instrument.lvclass.vi"("error in (no error)"=w8767, "Instrument.lvclass"=w8769, "S4ACS_GUI in"=w8768) -> ("error out"=w8766:errorcluster, "S4ACS_GUI out"=w8764:refnum<class "S4GUI.lvclass">)  [unwired: 7 in]
      }
      event "GFOC_stop": Value Change {
        n3533 = event-data() -> ()  [unwired: 1 in, 4 out]
        n3534 = call "Read Instrument.lvclass.vi"("error in (no error)"=w8802, "S4ACS_GUI in"=w8803) -> ("error out"=w8800:errorcluster, "Instrument.lvclass"=w8801:refnum<class "Instrument.lvclass">, "S4ACS_GUI out"=w8787:refnum<class "S4GUI.lvclass">)  [unwired: 7 in]
        n3535 = call "Read GFOC.vi"("error in (no error)"=w8800, "Instrument in"=w8801) -> ("error out"=w8796:errorcluster, "Opt_Continuous.lvclass"=w8799:refnum<class "Opt_Continuous.lvclass">, "Instrument out"=w8790:refnum<class "Instrument.lvclass">)  [unwired: 7 in]
        n3536 = call-dynamic "Read State Machine.vi"("error in (no error)"=w8796, "Device in"=w8799) -> ("error out"=w8795:errorcluster, "State Machine.lvclass"=w8798:refnum<class "State Machine.lvclass">, "Device out"=w8792:refnum<class "Opt_Continuous.lvclass">)  [unwired: 7 in]
        n3537 = call "Next State.vi"("error in (no error)"=w8795, "New_State"=10, "State Machine in"=w8798) -> ("error out"=w8794:errorcluster, "State Machine out"=w8793:refnum<class "State Machine.lvclass">)  [unwired: 7 in]
        n3538 = call-dynamic "Write State Machine.vi"("error in (no error)"=w8794, "State Machine.lvclass"=w8793, "Device in"=w8792) -> ("error out"=w8789:errorcluster, "Device out"=w8791:refnum<class "Opt_Continuous.lvclass">)  [unwired: 7 in]
        n3539 = call "Write GFOC.vi"("error in (no error)"=w8789, "Opt_Continuous.lvclass"=w8791, "Instrument in"=w8790) -> ("error out"=w8786:errorcluster, "Instrument out"=w8788:refnum<class "Instrument.lvclass">)  [unwired: 7 in]
        n3540 = call "Write Instrument.lvclass.vi"("error in (no error)"=w8786, "Instrument.lvclass"=w8788, "S4ACS_GUI in"=w8787) -> ("error out"=w8785:errorcluster, "S4ACS_GUI out"=w8784:refnum<class "S4GUI.lvclass">)  [unwired: 7 in]
      }
      event "GFOC_init": Value Change {
        n3541 = event-data() -> ()  [unwired: 1 in, 4 out]
        n3542 = call "Read Instrument.lvclass.vi"("error in (no error)"=w8822, "S4ACS_GUI in"=w8823) -> ("error out"=w8820:errorcluster, "Instrument.lvclass"=w8821:refnum<class "Instrument.lvclass">, "S4ACS_GUI out"=w8807:refnum<class "S4GUI.lvclass">)  [unwired: 7 in]
        n3543 = call "Read GFOC.vi"("error in (no error)"=w8820, "Instrument in"=w8821) -> ("error out"=w8816:errorcluster, "Opt_Continuous.lvclass"=w8819:refnum<class "Opt_Continuous.lvclass">, "Instrument out"=w8810:refnum<class "Instrument.lvclass">)  [unwired: 7 in]
        n3544 = call-dynamic "Read State Machine.vi"("error in (no error)"=w8816, "Device in"=w8819) -> ("error out"=w8815:errorcluster, "State Machine.lvclass"=w8818:refnum<class "State Machine.lvclass">, "Device out"=w8812:refnum<class "Opt_Continuous.lvclass">)  [unwired: 7 in]
        n3545 = call "Next State.vi"("error in (no error)"=w8815, "New_State"=30, "State Machine in"=w8818) -> ("error out"=w8814:errorcluster, "State Machine out"=w8813:refnum<class "State Machine.lvclass">)  [unwired: 7 in]
        n3546 = call-dynamic "Write State Machine.vi"("error in (no error)"=w8814, "State Machine.lvclass"=w8813, "Device in"=w8812) -> ("error out"=w8809:errorcluster, "Device out"=w8811:refnum<class "Opt_Continuous.lvclass">)  [unwired: 7 in]
        n3547 = call "Write GFOC.vi"("error in (no error)"=w8809, "Opt_Continuous.lvclass"=w8811, "Instrument in"=w8810) -> ("error out"=w8806:errorcluster, "Instrument out"=w8808:refnum<class "Instrument.lvclass">)  [unwired: 7 in]
        n3548 = call "Write Instrument.lvclass.vi"("error in (no error)"=w8806, "Instrument.lvclass"=w8808, "S4ACS_GUI in"=w8807) -> ("error out"=w8805:errorcluster, "S4ACS_GUI out"=w8804:refnum<class "S4GUI.lvclass">)  [unwired: 7 in]
      }
      event "CALW_target": Value Change {
        n3549 = event-data() -> ("NewVal"=w8833:dbl)  [unwired: 1 in, 3 out]
        n3550 = call "Read Instrument.lvclass.vi"("error in (no error)"=w8837, "S4ACS_GUI in"=w8838) -> ("error out"=w8835:errorcluster, "Instrument.lvclass"=w8836:refnum<class "Instrument.lvclass">, "S4ACS_GUI out"=w8827:refnum<class "S4GUI.lvclass">)  [unwired: 7 in]
        n3551 = call "Read CALW.vi"("error in (no error)"=w8835, "Instrument in"=w8836) -> ("error out"=w8832:errorcluster, "Opt_Selector.lvclass"=w8834:refnum<class "Opt_Selector.lvclass">, "Instrument out"=w8830:refnum<class "Instrument.lvclass">)  [unwired: 7 in]
        n3552 = call "Write target.vi"("error in (no error)"=w8832, "target"=w8833, "Optics in"=w8834) -> ("error out"=w8829:errorcluster, "Optics out"=w8831:refnum<class "Opt_Selector.lvclass">)  [unwired: 7 in]
        n3553 = call "Write CALW.vi"("error in (no error)"=w8829, "Opt_Selector.lvclass"=w8831, "Instrument in"=w8830) -> ("error out"=w8826:errorcluster, "Instrument out"=w8828:refnum<class "Instrument.lvclass">)  [unwired: 7 in]
        n3554 = call "Write Instrument.lvclass.vi"("error in (no error)"=w8826, "Instrument.lvclass"=w8828, "S4ACS_GUI in"=w8827) -> ("error out"=w8825:errorcluster, "S4ACS_GUI out"=w8824:refnum<class "S4GUI.lvclass">)  [unwired: 7 in]
      }
      event "CALW_set": Value Change {
        n3555 = event-data() -> ()  [unwired: 1 in, 4 out]
        n3556 = call "Read Instrument.lvclass.vi"("error in (no error)"=w8857, "S4ACS_GUI in"=w8858) -> ("error out"=w8855:errorcluster, "Instrument.lvclass"=w8856:refnum<class "Instrument.lvclass">, "S4ACS_GUI out"=w8843:refnum<class "S4GUI.lvclass">)  [unwired: 7 in]
        n3557 = call "Read CALW.vi"("error in (no error)"=w8855, "Instrument in"=w8856) -> ("error out"=w8852:errorcluster, "Opt_Selector.lvclass"=w8854:refnum<class "Opt_Selector.lvclass">, "Instrument out"=w8846:refnum<class "Instrument.lvclass">)  [unwired: 7 in]
        n3558 = call-dynamic "Read State Machine.vi"("error in (no error)"=w8852, "Device in"=w8854) -> ("error out"=w8851:errorcluster, "State Machine.lvclass"=w8840:refnum<class "State Machine.lvclass">, "Device out"=w8848:refnum<class "Opt_Selector.lvclass">)  [unwired: 7 in]
        n3559 = call "Next State.vi"("error in (no error)"=w8851, "New_State"=1, "State Machine in"=w8840) -> ("error out"=w8850:errorcluster, "State Machine out"=w8849:refnum<class "State Machine.lvclass">)  [unwired: 7 in]
        n3560 = call-dynamic "Write State Machine.vi"("error in (no error)"=w8850, "State Machine.lvclass"=w8849, "Device in"=w8848) -> ("error out"=w8845:errorcluster, "Device out"=w8847:refnum<class "Opt_Selector.lvclass">)  [unwired: 7 in]
        n3561 = call "Write CALW.vi"("error in (no error)"=w8845, "Opt_Selector.lvclass"=w8847, "Instrument in"=w8846) -> ("error out"=w8842:errorcluster, "Instrument out"=w8844:refnum<class "Instrument.lvclass">)  [unwired: 7 in]
        n3562 = call "Write Instrument.lvclass.vi"("error in (no error)"=w8842, "Instrument.lvclass"=w8844, "S4ACS_GUI in"=w8843) -> ("error out"=w8841:errorcluster, "S4ACS_GUI out"=w8839:refnum<class "S4GUI.lvclass">)  [unwired: 7 in]
      }
      event "CALW_stop": Value Change {
        n3563 = event-data() -> ()  [unwired: 1 in, 4 out]
        n3564 = call "Read Instrument.lvclass.vi"("error in (no error)"=w8877, "S4ACS_GUI in"=w8878) -> ("error out"=w8875:errorcluster, "Instrument.lvclass"=w8876:refnum<class "Instrument.lvclass">, "S4ACS_GUI out"=w8862:refnum<class "S4GUI.lvclass">)  [unwired: 7 in]
        n3565 = call "Read CALW.vi"("error in (no error)"=w8875, "Instrument in"=w8876) -> ("error out"=w8871:errorcluster, "Opt_Selector.lvclass"=w8874:refnum<class "Opt_Selector.lvclass">, "Instrument out"=w8865:refnum<class "Instrument.lvclass">)  [unwired: 7 in]
        n3566 = call-dynamic "Read State Machine.vi"("error in (no error)"=w8871, "Device in"=w8874) -> ("error out"=w8870:errorcluster, "State Machine.lvclass"=w8873:refnum<class "State Machine.lvclass">, "Device out"=w8867:refnum<class "Opt_Selector.lvclass">)  [unwired: 7 in]
        n3567 = call "Next State.vi"("error in (no error)"=w8870, "New_State"=10, "State Machine in"=w8873) -> ("error out"=w8869:errorcluster, "State Machine out"=w8868:refnum<class "State Machine.lvclass">)  [unwired: 7 in]
        n3568 = call-dynamic "Write State Machine.vi"("error in (no error)"=w8869, "State Machine.lvclass"=w8868, "Device in"=w8867) -> ("error out"=w8864:errorcluster, "Device out"=w8866:refnum<class "Opt_Selector.lvclass">)  [unwired: 7 in]
        n3569 = call "Write CALW.vi"("error in (no error)"=w8864, "Opt_Selector.lvclass"=w8866, "Instrument in"=w8865) -> ("error out"=w8861:errorcluster, "Instrument out"=w8863:refnum<class "Instrument.lvclass">)  [unwired: 7 in]
        n3570 = call "Write Instrument.lvclass.vi"("error in (no error)"=w8861, "Instrument.lvclass"=w8863, "S4ACS_GUI in"=w8862) -> ("error out"=w8860:errorcluster, "S4ACS_GUI out"=w8859:refnum<class "S4GUI.lvclass">)  [unwired: 7 in]
      }
      event "CALW_init": Value Change {
        n3571 = event-data() -> ()  [unwired: 1 in, 4 out]
        n3572 = call "Read Instrument.lvclass.vi"("error in (no error)"=w8897, "S4ACS_GUI in"=w8898) -> ("error out"=w8895:errorcluster, "Instrument.lvclass"=w8896:refnum<class "Instrument.lvclass">, "S4ACS_GUI out"=w8882:refnum<class "S4GUI.lvclass">)  [unwired: 7 in]
        n3573 = call "Read CALW.vi"("error in (no error)"=w8895, "Instrument in"=w8896) -> ("error out"=w8891:errorcluster, "Opt_Selector.lvclass"=w8894:refnum<class "Opt_Selector.lvclass">, "Instrument out"=w8885:refnum<class "Instrument.lvclass">)  [unwired: 7 in]
        n3574 = call-dynamic "Read State Machine.vi"("error in (no error)"=w8891, "Device in"=w8894) -> ("error out"=w8890:errorcluster, "State Machine.lvclass"=w8893:refnum<class "State Machine.lvclass">, "Device out"=w8887:refnum<class "Opt_Selector.lvclass">)  [unwired: 7 in]
        n3575 = call "Next State.vi"("error in (no error)"=w8890, "New_State"=30, "State Machine in"=w8893) -> ("error out"=w8889:errorcluster, "State Machine out"=w8888:refnum<class "State Machine.lvclass">)  [unwired: 7 in]
        n3576 = call-dynamic "Write State Machine.vi"("error in (no error)"=w8889, "State Machine.lvclass"=w8888, "Device in"=w8887) -> ("error out"=w8884:errorcluster, "Device out"=w8886:refnum<class "Opt_Selector.lvclass">)  [unwired: 7 in]
        n3577 = call "Write CALW.vi"("error in (no error)"=w8884, "Opt_Selector.lvclass"=w8886, "Instrument in"=w8885) -> ("error out"=w8881:errorcluster, "Instrument out"=w8883:refnum<class "Instrument.lvclass">)  [unwired: 7 in]
        n3578 = call "Write Instrument.lvclass.vi"("error in (no error)"=w8881, "Instrument.lvclass"=w8883, "S4ACS_GUI in"=w8882) -> ("error out"=w8880:errorcluster, "S4ACS_GUI out"=w8879:refnum<class "S4GUI.lvclass">)  [unwired: 7 in]
      }
      event "ASEL_target": Value Change {
        n3579 = event-data() -> ("NewVal"=w8908:dbl)  [unwired: 1 in, 3 out]
        n3580 = call "Read Instrument.lvclass.vi"("error in (no error)"=w8912, "S4ACS_GUI in"=w8913) -> ("error out"=w8910:errorcluster, "Instrument.lvclass"=w8911:refnum<class "Instrument.lvclass">, "S4ACS_GUI out"=w8902:refnum<class "S4GUI.lvclass">)  [unwired: 7 in]
        n3581 = call "Read ASEL.vi"("error in (no error)"=w8910, "Instrument in"=w8911) -> ("error out"=w8907:errorcluster, "Opt_Selector.lvclass"=w8909:refnum<class "Opt_Selector.lvclass">, "Instrument out"=w8905:refnum<class "Instrument.lvclass">)  [unwired: 7 in]
        n3582 = call "Write target.vi"("error in (no error)"=w8907, "target"=w8908, "Optics in"=w8909) -> ("error out"=w8904:errorcluster, "Optics out"=w8906:refnum<class "Opt_Selector.lvclass">)  [unwired: 7 in]
        n3583 = call "Write ASEL.vi"("error in (no error)"=w8904, "Opt_Selector.lvclass"=w8906, "Instrument in"=w8905) -> ("error out"=w8901:errorcluster, "Instrument out"=w8903:refnum<class "Instrument.lvclass">)  [unwired: 7 in]
        n3584 = call "Write Instrument.lvclass.vi"("error in (no error)"=w8901, "Instrument.lvclass"=w8903, "S4ACS_GUI in"=w8902) -> ("error out"=w8900:errorcluster, "S4ACS_GUI out"=w8899:refnum<class "S4GUI.lvclass">)  [unwired: 7 in]
      }
      event "ASEL_set": Value Change {
        n3585 = event-data() -> ()  [unwired: 1 in, 4 out]
        n3586 = call "Read Instrument.lvclass.vi"("error in (no error)"=w8932, "S4ACS_GUI in"=w8933) -> ("error out"=w8930:errorcluster, "Instrument.lvclass"=w8931:refnum<class "Instrument.lvclass">, "S4ACS_GUI out"=w8918:refnum<class "S4GUI.lvclass">)  [unwired: 7 in]
